vi "Diff Test.vi"() -> ()   [LabVIEW 2017]
doc: "Shows the use of JSON Difference in JSONtext."
uses:
  JSONtext.lvlib
  <vilib>/addons/_JKI Toolkits/Caraya/classes/Assert/Assert.lvclass
  <vilib>/addons/_JKI Toolkits/Caraya/classes/Test/Test.lvclass
panel:
  out "<JSON> 2":string caption="Changes (Second from First)"
  out "<JSON>":string caption="Changes (First from Second)"
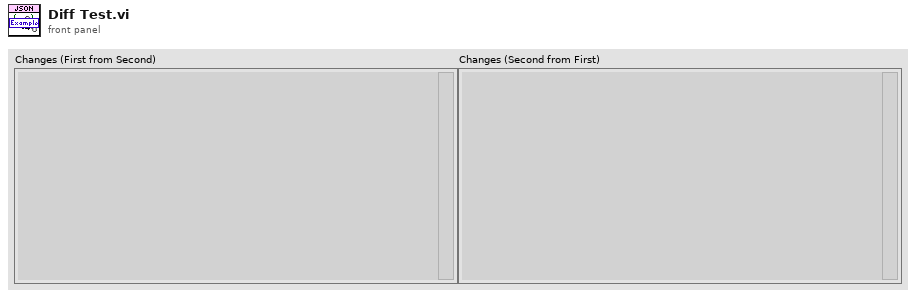
[diagram p1: front panel]
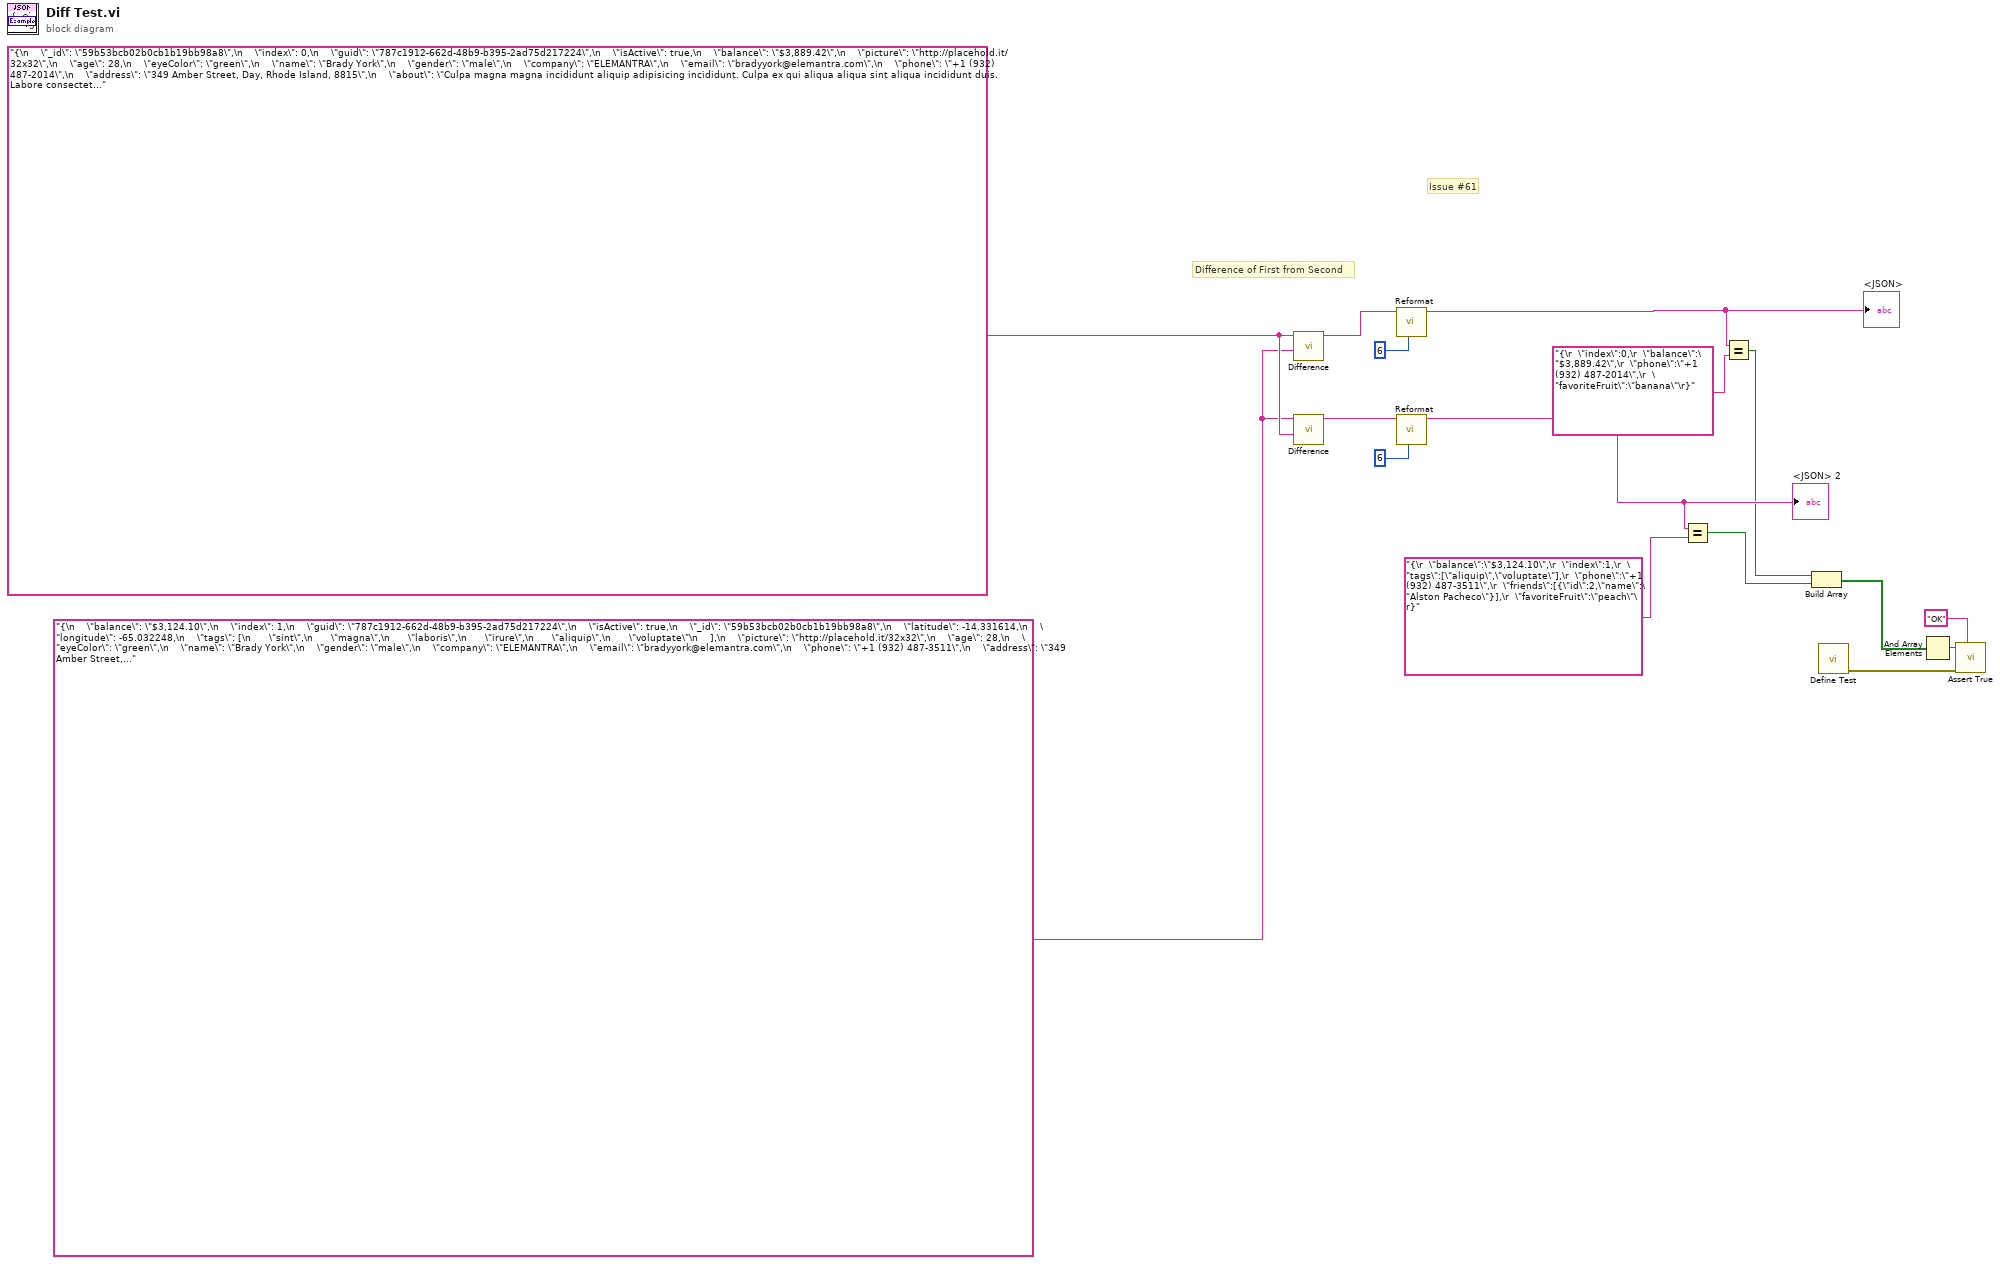
[diagram p0: block diagram]
diagram:
  w11 = "{\n    \"balance\": \"$3,124.10\",\n    \"index\": 1,\n    \"guid\": \"787c1912-662d-48b9-b395-2ad75d217224\",\n    \"isActive\": true,\n    \"_id\": \"59b53bcb02b0cb1b19bb98a8\",\n    \"latitude\": -14.331614,\n    \"longitude\": -65.032248,\n    \"tags\": [\n      \"sint\",\n      \"magna\",\n      \"laboris\",\n      \"irure\",\n      \"aliquip\",\n      \"voluptate\"\n    ],\n    \"picture\": \"http://placehold.it/32x32\",\n    \"age\": 28,\n    \"eyeColor\": \"green\",\n    \"name\": \"Brady York\",\n    \"gender\": \"male\",\n    \"company\": \"ELEMANTRA\",\n    \"email\": \"bradyyork@elemantra.com\",\n    \"phone\": \"+1 (932) 487-3511\",\n    \"address\": \"349 Amber Street, Day, Rhode Island, 8815\",\n    \"about\": \"Culpa magna magna incididunt aliquip adipisicing incididunt. Culpa ex qui aliqua aliqua sint aliqua incididunt duis. Labore consectetur in pariatur qui anim reprehenderit duis.\\r\\n\",\n    \"registered\": \"2014-10-21T08:11:24 -01:00\",\n    \"friends\": [\n      {\n        \"id\": 0,\n        \"name\": \"Magdalena Stanley\"\n      },\n      {\n        \"id\": 1,\n        \"name\": \"Gill Alvarez\"\n      },\n      {\n        \"id\": 2,\n        \"name\": \"Alston Pacheco\"\n      }\n    ],\n    \"greeting\": \"Hello, Brady York! You have 8 unread messages.\",\n    \"favoriteFruit\": \"peach\"\n  }" ("Second")
  w12 = "{\n    \"_id\": \"59b53bcb02b0cb1b19bb98a8\",\n    \"index\": 0,\n    \"guid\": \"787c1912-662d-48b9-b395-2ad75d217224\",\n    \"isActive\": true,\n    \"balance\": \"$3,889.42\",\n    \"picture\": \"http://placehold.it/32x32\",\n    \"age\": 28,\n    \"eyeColor\": \"green\",\n    \"name\": \"Brady York\",\n    \"gender\": \"male\",\n    \"company\": \"ELEMANTRA\",\n    \"email\": \"bradyyork@elemantra.com\",\n    \"phone\": \"+1 (932) 487-2014\",\n    \"address\": \"349 Amber Street, Day, Rhode Island, 8815\",\n    \"about\": \"Culpa magna magna incididunt aliquip adipisicing incididunt. Culpa ex qui aliqua aliqua sint aliqua incididunt duis. Labore consectetur in pariatur qui anim reprehenderit duis.\\r\\n\",\n    \"registered\": \"2014-10-21T08:11:24 -01:00\",\n    \"latitude\": -14.331614,\n    \"longitude\": -65.032248,\n    \"tags\": [\n      \"sint\",\n      \"magna\",\n      \"laboris\",\n      \"irure\"\n    ],\n    \"friends\": [\n      {\n      \"name\": \"Magdalena Stanley\", \"id\": 0\n      },\n      {\n        \"id\": 1,\n        \"name\":   \"Gill Alvarez\"   \n\n      }\n    ],\n    \"greeting\": \"Hello, Brady York! You have 8 unread messages.\",\n    \"favoriteFruit\": \"banana\"\n  }" ("First")
  # "Issue #61"
  # "Difference of First from Second"
  n1 = call "Difference.vi"("Compare to this JSON Object"=w11, "JSON Object"=w12) -> ("<JSON>"=w16:string)  [unwired: 7 in, 1 out]
  n2 = call "Difference.vi"("Compare to this JSON Object"=w12, "JSON Object"=w11) -> ("<JSON>"=w13:string)  [unwired: 7 in, 1 out]
  n3 = call "Reformat.vi"("Pretty Print Levels"=6, "JSON"=w16) -> ("<JSON>First JSON Value\n\n<JSON>"=w10:string)  [unwired: 6 in, 3 out]
  "<JSON>" <- w10
  n4 = call "Reformat.vi"("Pretty Print Levels"=6, "JSON"=w13) -> ("<JSON>First JSON Value\n\n<JSON>"=w8:string)  [unwired: 6 in, 3 out]
  "<JSON> 2" <- w8
  n5 = Equal?(x=w8, y="{\r  \"balance\":\"$3,124.10\",\r  \"index\":1,\r  \"tags\":[\"aliquip\",\"voluptate\"],\r  \"phone\":\"+1 (932) 487-3511\",\r  \"friends\":[{\"id\":2,\"name\":\"Alston Pacheco\"}],\r  \"favoriteFruit\":\"peach\"\r}" ("<JSON> 2")) -> (x = y?=w2:bool)
  n6 = Equal?(x=w10, y="{\r  \"index\":0,\r  \"balance\":\"$3,889.42\",\r  \"phone\":\"+1 (932) 487-2014\",\r  \"favoriteFruit\":\"banana\"\r}" ("<JSON>")) -> (x = y?=w3:bool)
  n7 = Build Array(w3, w2) -> (w1:bool[])
  n8 = call <vilib>:"Define Test.vi"() -> ("error out"=w4:errorcluster)  [unwired: 11 in]
  n9 = And Array Elements(Boolean array=w1) -> (logical AND=w6:bool)
  n10 = call <vilib>:"Assert True.vi"("Label"="OK", "error in (no error)"=w4, "True?"=w6) -> ()  [unwired: 8 in, 1 out]
